vi "WritePinMode.vi"(8 "error in (no error)":errorcluster, 9 "Pin Mode":T1 items=["Input", "Output"], 10 "Pin":T2=2 items=["D2"=2, "D3"=3, "D4"=4, "D5"=5, "D6"=6, "D7"=7, "D8"=8, "D9"=9, "A0"=14, "A1"=15, "A2"=16, "A3"=17], 11 "GrovePi in":refnum<class "GrovePi.lvclass">) -> (0 "error out":errorcluster, 3 "GrovePi out":refnum<class "GrovePi.lvclass">)   [LabVIEW 2014, in "GrovePi.lvclass"]
doc: "Sets the Pin Mode (input or output) of a Pin on the GrovePi."
uses:
  GrovePi.lvclass
  Pin.ctl
  PinMode.ctl
  Command.ctl
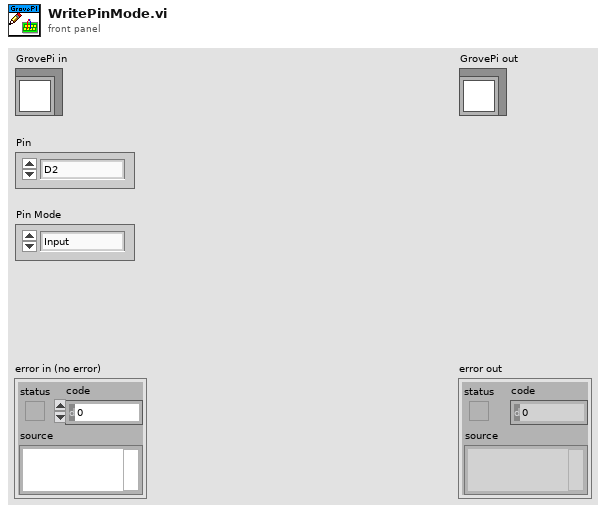
[diagram p1: front panel]
types:
  T1 = typedef "GrovePi.lvclass/PinMode.ctl" = u8
  T2 = typedef "GrovePi.lvclass/Pin.ctl" = u8
  T3 = typedef "GrovePi.lvclass/Command.ctl" = u8
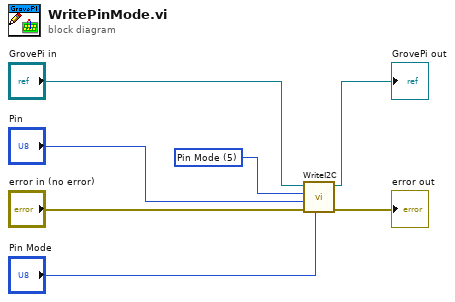
[diagram p0: block diagram]
diagram:
  w4 = T3 5 items=["Digital Read"=1, "Digital Write"=2, "Analog Read"=3, "Analog Write"=4, "Pin Mode"=5, "Ultrasonic Read"=7, "Version"=8, "Dust Sensor Read"=10, "Encoder Read"=11, "Flow Read"=12, "Flow Disabled"=13, "Dust Sensor Enable"=14, "Dust Sensor Disable"=15, "Encoder Enable"=16, "Encoder Disable"=17, "Flow Enable"=18, "Accelerometer Read"=20, "RTC Read"=30, "DHT Read"=40] ("Command")
  n1 = call "WriteI2C.vi"("Byte 2"="Pin Mode", "error in (no error)"="error in (no error)", "Pin"="Pin", "Command"=w4, "GrovePi in"="GrovePi in") -> ("error out"=→"error out":errorcluster, "GrovePi out"=→"GrovePi out":refnum<class "GrovePi.lvclass">)  [unwired: 4 in, 1 out]
